vi "LDO_Update_Intellifaucet_Parameters.vi"(7 "FVIR?":bool, 8 "error in (no error)":errorcluster, 9 "Valve % Open - Automatic Mode":dbl=15.0 min=15.0 max=100.0, 10 "Temp (°F) - Automatic Mode":dbl=32.0 min=32.0 max=203.0, 11 "Modbus Input":refnum<queue>) -> (0 "error out":errorcluster, 3 "dup Message Queue":refnum<queue>)   [LabVIEW 2023]
uses:
  Message Queue/Message Cluster.ctl
  Message Queue/Enqueue Message (Single).vi
  Message Queue/Message Queue.lvlib
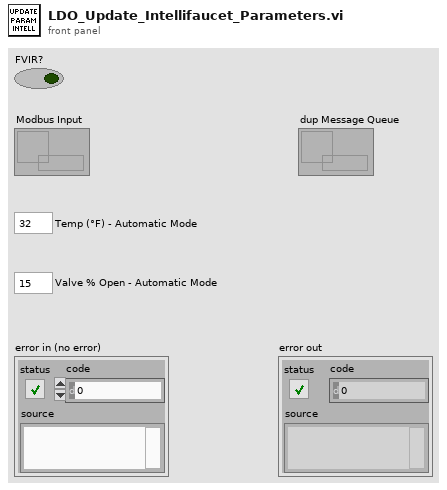
[diagram p1: front panel]
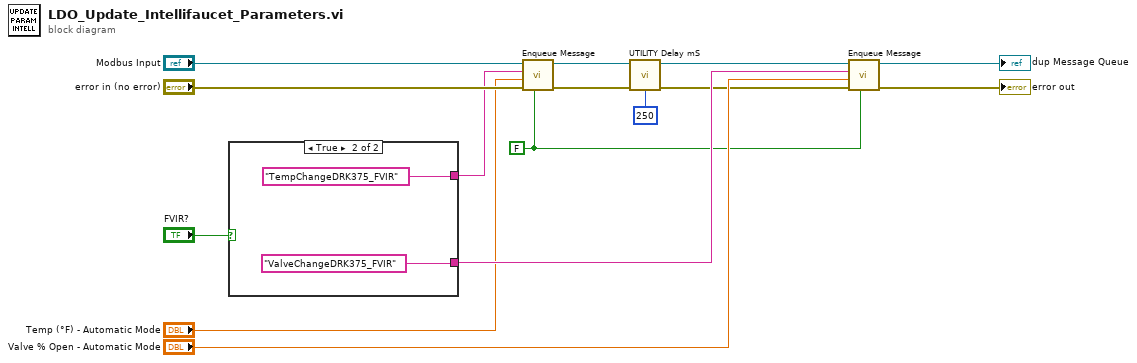
[diagram p0: block diagram]
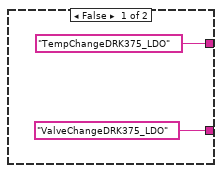
[diagram p2: hidden frame]
diagram:
  w4 = FALSE ("Priority Message? (F)")
  n1 = case shown="True" "FVIR?" {
    tunnel: ["ValveChangeDRK375_LDO" ("Message") "ValveChangeDRK375_FVIR" ("Message")] -> w11
    tunnel: ["TempChangeDRK375_LDO" ("Message") "TempChangeDRK375_FVIR" ("Message")] -> w8
    frame False {
    }
    frame True {
    }
  }
  n2 = call-poly "Enqueue Message.vi"("Priority Message? (F)"=w4, "error in (no error)"="error in (no error)", "Message Data"="Temp (°F) - Automatic Mode", "Message"=w8, "Message Queue"="Modbus Input") -> ("error out"=w2:errorcluster, "dup Message Queue"=w5:refnum<queue>)  [unwired: 5 in]
  n3 = call "UTILITY Delay mS.vi"("Error In"=w2, "milliseconds to wait"=u32 250) -> ("Error Out"=w1:errorcluster)  [unwired: 13 in]
  n4 = call-poly "Enqueue Message.vi"("Priority Message? (F)"=w4, "error in (no error)"=w1, "Message Data"="Valve % Open - Automatic Mode", "Message"=w11, "Message Queue"=w5) -> ("error out"=→"error out":errorcluster, "dup Message Queue"=→"dup Message Queue":refnum<queue>)  [unwired: 5 in]
